vi "Tag Size.vi"(8 "error in (no error)":errorcluster, 11 "IFD_Tag in":refnum<class "IFD_Tag.lvclass">) -> (0 "error out":errorcluster, 1 "Reference?":bool, 2 "Byte Count":u32, 3 "IFD_Tag out":refnum<class "IFD_Tag.lvclass">)   [LabVIEW 2016, in "IFD_Tag.lvclass"]
uses:
  IFD_Tag.lvclass
  IFD_Tag.lvclass/IFD_Tag.ctl
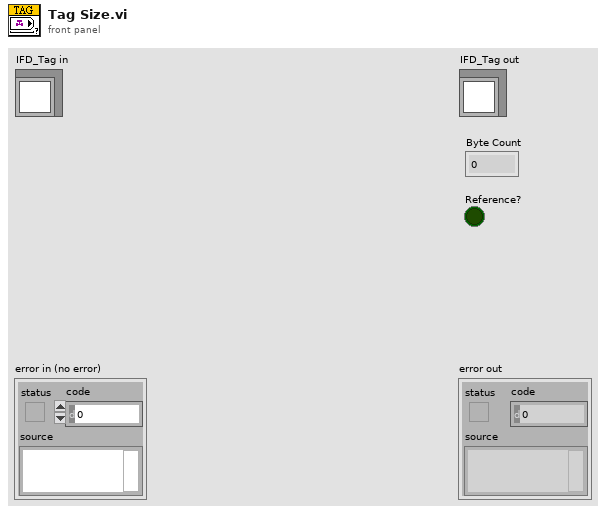
[diagram p1: front panel]
types:
  T1 = enum16{"Undefined(DO NOT USE)", "U8", "ASCII", "U16", "U32", "RATIONAL", "I8", "Undefined 8 bit", "I16", "I32", "SRATIONAL", "SGL", "DBL"}
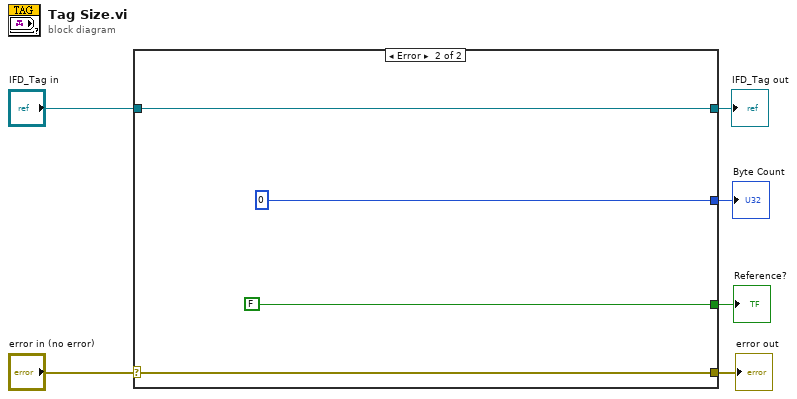
[diagram p0: block diagram]
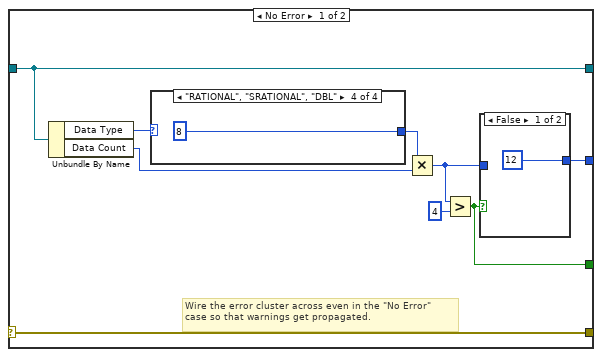
[diagram p2: hidden frame]
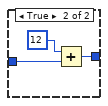
[diagram p3: hidden frame]
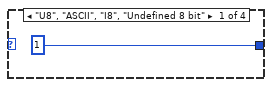
[diagram p4: hidden frame]
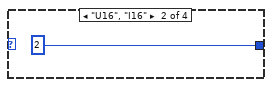
[diagram p5: hidden frame]
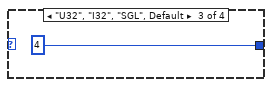
[diagram p6: hidden frame]
diagram:
  n1 = case shown="Error" "error in (no error)" {
    selector: "error in (no error)" -> [w15 w27]
    tunnel: [w15 w27] -> w5
    tunnel: [w14 w26] -> w3
    tunnel: "IFD_Tag in" -> [w14 w26]
    tunnel: [w8 u32 0] -> w2
    tunnel: [w7 FALSE] -> w1
    frame No Error {
      # "Wire the error cluster across even in the \"No Error\"\ncase so that warnings get propagated."
      n2 = Unbundle By Name(w14) -> ("Data Type"=w13:T1, "Data Count"=w11:u32)
      n3 = case shown="\"RATIONAL\", \"SRATIONAL\", \"DBL\"" w13 {
        tunnel: [u32 1 u32 2 u32 4 u32 8] -> w12
        frame "U8", "ASCII", "I8", "Undefined 8 bit" {
        }
        frame "U16", "I16" {
        }
        frame "U32", "I32", "SGL", Default {
        }
        frame "RATIONAL", "SRATIONAL", "DBL" {
        }
      }
      n4 = Multiply(x=w12, y=w11) -> (x*y=w9:u32)
      n5 = Greater?(x=w9, y=u32 4) -> (0:w7:bool)
      n6 = case shown="False" w7 {
        tunnel: w9 -> [_ w18]
        tunnel: [u32 12 w17] -> w8
        frame False {
        }
        frame True {
          n7 = Add(x=u32 12, y=w18) -> (x+y=w17:u32)
        }
      }
    }
    frame Error {
    }
  }
  "error out" <- w5
  "IFD_Tag out" <- w3
  "Byte Count" <- w2
  "Reference?" <- w1
